vi "CalcTrigAbsAngle.vi"(10 "Point 2":T1 {"North" format="%#_10f"; "East" format="%#_8f"}, 11 "Point 1":T1 {"North" format="%#_10f"; "East" format="%#_8f"}) -> (3 "Angle between points (rad)":dbl)   [LabVIEW 2013]
doc: "Takes two points and returns their angle relative to trig zero. All angles represented in positive radians.\nPoint 1 is the origin, from which Point 2 forms the ray that is evaluated against trig zero."
uses:
  Data/TypeDefs/UTM Location.ctl
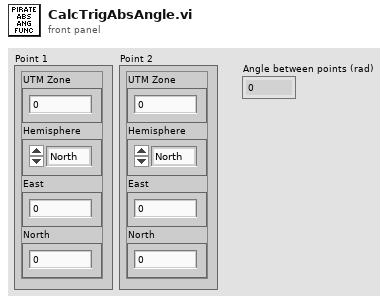
[diagram p1: front panel]
types:
  T1 = typedef "UTM Location.ctl" = cluster{"UTM Zone":dbl, "Hemisphere":enum16{"North", "South"}, "East":dbl, "North":dbl}
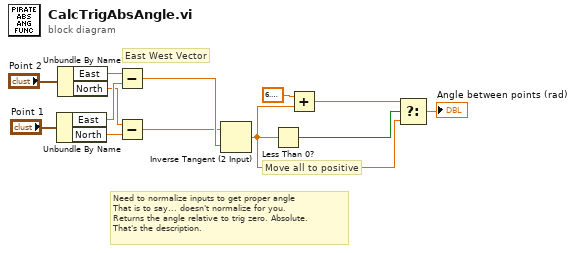
[diagram p0: block diagram]
diagram:
  # "Move all to positive"
  # "East West Vector"
  # "Need to normalize inputs to get proper angle\nThat is to say... doesn't normalize for you.\nReturns the angle relative to trig zero. Absolute.\nThat's the description."
  n1 = Unbundle By Name("Point 1") -> ("East"=w10:dbl, "North"=w8:dbl)
  n2 = Unbundle By Name("Point 2") -> ("East"=w11:dbl, "North"=w9:dbl)
  n3 = Subtract(x=w11, y=w10) -> (x-y=w4:dbl)
  n4 = Subtract(x=w9, y=w8) -> (x-y=w3:dbl)
  n5 = Inverse Tangent (2 Input)(1:w4, 2:w3) -> (0:w6:dbl)
  n6 = Less Than 0?(x=w6) -> (x < 0?=w7:bool)
  n7 = Add(x=6.283185307179586, y=w6) -> (x+y=w1:dbl)
  n8 = Select(t=w1, s=w7, f=w6) -> (s? t:f=→"Angle between points (rad)":dbl)
